vi "Core.vi"(8 "error in (no error)":errorcluster, 11 "Scenarios Class in":refnum<class "Scenarios Class.lvclass">) -> (0 "error out":errorcluster, 3 "Scenarios Class out":refnum<class "Scenarios Class.lvclass">)   [LabVIEW 2020, in "SECS Scenarios.lvlib" / "Scenarios Class.lvclass"]
uses:
  Scenarios Class.lvclass
  Scenarios Class.lvclass/Scenarios Class.ctl
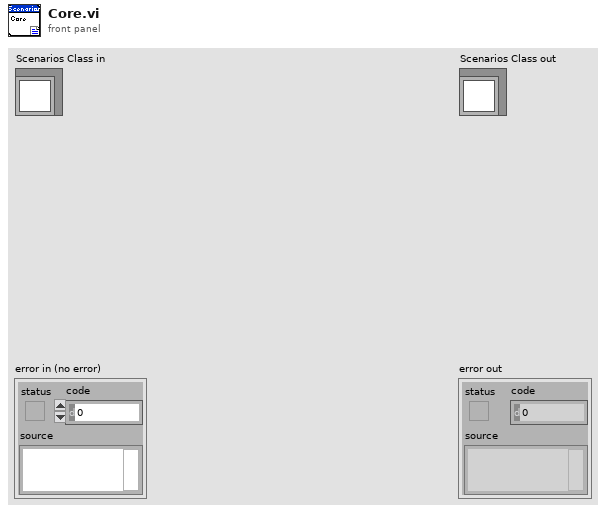
[diagram p1: front panel]
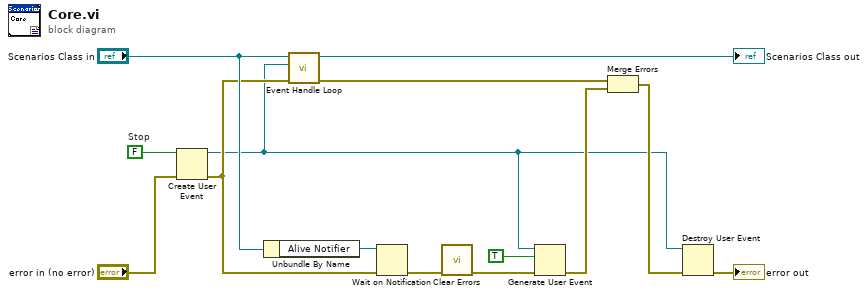
[diagram p0: block diagram]
diagram:
  w12 = FALSE  # Stop
  n1 = Create User Event(user event datatype=w12, error in="error in (no error)") -> (user event=w1:refnum<user-event>, error out=w10:errorcluster)
  n2 = Unbundle By Name("Scenarios Class in") -> ("Alive Notifier"=w14:refnum<notifier>)
  n3 = call "Event Handle Loop.vi"("error in (no error)"=w10, "Stop User Event"=w1, "Scenarios Class in"="Scenarios Class in") -> ("error out"=w6:errorcluster, "Scenarios Class out"=→"Scenarios Class out":refnum<class "Scenarios Class.lvclass">)  [unwired: 7 in]
  n4 = Wait on Notification(notifier=w14, error in (no error)=w10) -> (error out=w9:errorcluster)  [unwired: 2 in, 3 out]
  n5 = call <vilib>:"Clear Errors.vi"("error in (no error)"=w9) -> ("error out"=w8:errorcluster)  [unwired: 5 in, 1 out]
  n6 = Generate User Event(user event=w1, event data cluster=TRUE ("event data"), error in=w8) -> (error out=w5:errorcluster)  [unwired: 1 in, 1 out]
  n7 = Merge Errors(w6, w5) -> (w3:errorcluster)
  n8 = Destroy User Event(user event=w1, error in=w3) -> (error out=→"error out":errorcluster)
